vi "Temperature in File1.vi"(4 "Количество знаков после запятой":string, 5 "Ширина строки (в символах)":string, 6 "error in":errorcluster, 7 "Сопротивление при нуле":dbl, 8 "Значение температурного коэффициента":dbl, 9 "массив с сопротивлениями":dbl[](array[numeric]), 10 "Файл":refnum<file>, 11 "Количество датчиков":i32) -> (0 "Массив температур":dbl[](array[numeric]), 1 "error out":errorcluster, 3 "Файл 2":refnum<file>)   [LabVIEW 2018]
doc: "Переводит значение сопротивления в значения температуры. Значение температуры затем записываются в файл"
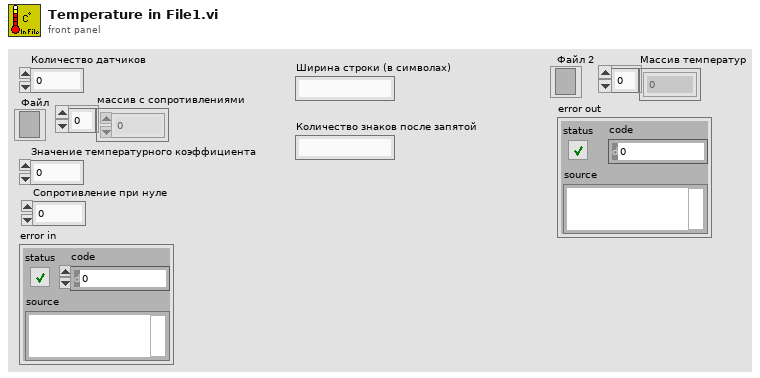
[diagram p1: front panel]
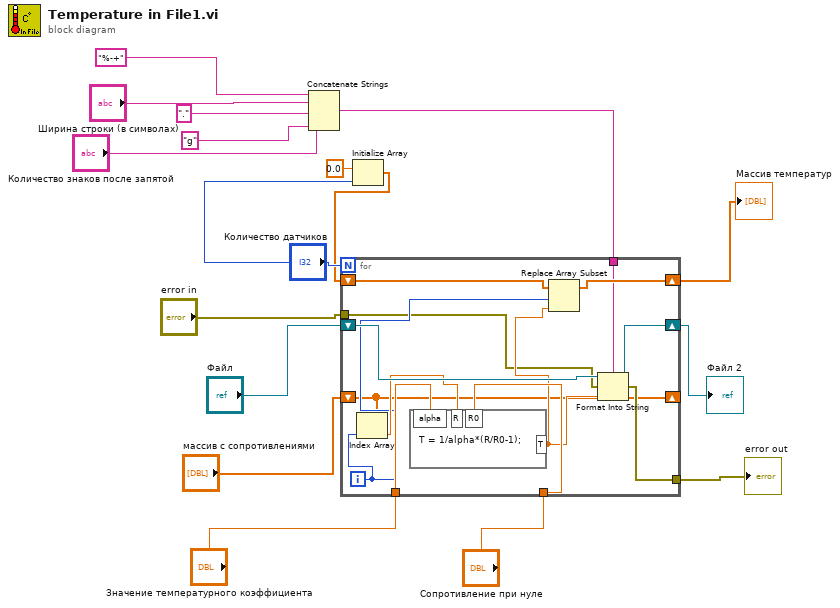
[diagram p0: block diagram]
diagram:
  n1 = Concatenate Strings("%-+" ("string"), "Ширина строки (в символах)", "." ("string"), "Количество знаков после запятой", "g" ("string")) -> (w1:string)
  n2 = Initialize Array(0.0 ("element"), "Количество датчиков") -> (w10:dbl[])
  n3 = for {
    N: "Количество датчиков" -> [_]
    tunnel: "Значение температурного коэффициента" -> [w30]
    tunnel: "Сопротивление при нуле" -> [w29]
    shift-right: [w27] -> w13
    shift-left: "Файл" -> [w28]
    tunnel: [w21] -> w8
    tunnel: "error in" -> [w20]
    shift-right: [w19] -> _
    shift-left: "массив с сопротивлениями" -> [w19]
    shift-right: [w22] -> w9
    shift-left: w10 -> [w25]
    tunnel: w1 -> [w18]
    i -> [w24]
    n4 = Index Array(array=w19, index=w24) -> (element=w26:dbl)
    n5 = formula code="T = 1/alpha*(R/R0-1);"("alpha"=w30, "R"=w26, "R0"=w29) -> ("T"=w23:dbl)
    n6 = Replace Array Subset(array=w25, new element=w23, index=w24) -> (w22:dbl[])
    n7 = Format Into String(format string=w18, initial string=w28, error in=w20, w23) -> (resulting string=w27:refnum<file>, error out=w21:errorcluster)
  }
  "Файл 2" <- w13
  "Массив температур" <- w9
  "error out" <- w8
